vi "dfd_Dummy_INT LatticeOneM.vi"(9 "k(m)":i16, 10 "w(m-1)":i32, 11 "x(m)":i32) -> (2 "w(m)":i32, 3 "x(m-1)":i32)   [LabVIEW 2017]
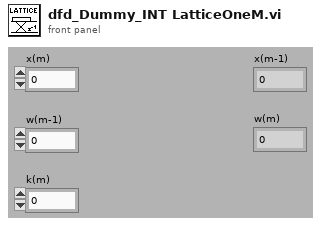
[diagram p1: front panel]
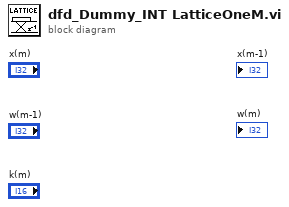
[diagram p0: block diagram]
diagram:
